vi "iHR550 Convert Axis.vi"(1 "iHR Current Values":T2={"iHR 550 Front Entrance"=0.0, "iHR550 Side Exit"=0.0, "iHR550 Wavelength"=897.9988, "iHR550 Exit Mirror"=2, "iHR550 Grating"="1", "Grating Index"=1} {"iHR550 Exit Mirror" items=["EntranceMirror", "ExitMirror", "Front", "Side"]}) -> (0 "Wavelengths (nm)":dbl[](array[numeric]))   [LabVIEW 2010]
uses:
  TypeDefs/iHR Current Values.ctl
  TypeDefs/iHR Instrument Parameters.ctl
panel:
  out "Tabellen-String":string
  out "l_p (nm)":dbl
  out "beta_lp (rad)":dbl
  out "H_Blp (mm)":dbl
  out "P_c":dbl
  out "beta_H (rad)":dbl
  out "beta_lc (rad)":dbl
  in  "Diffraction Order":i8=1
  in  "Grooves (1/mm)":i16[](array[numeric])=[1800, 600, 150]
  out "alpha_lc (rad)":dbl
  out "H_Blc (mm)":dbl
  out "L_H (mm)":dbl
  out "Inclination Angle (rad)":dbl
  out "Ebert Angle (rad)":dbl
  out "Pixel Width (mm)":dbl
  in  "iHR Instrument Parameters":T1={"Focal In (mm)"=546.0, "Focal Out (mm)"=568.72, "Pixel Width (µm)"=13.5, "Pixel Count"=2048, "Ebert Angle (°)"=6.498, "Inclination Angle (°)"=-2.35}
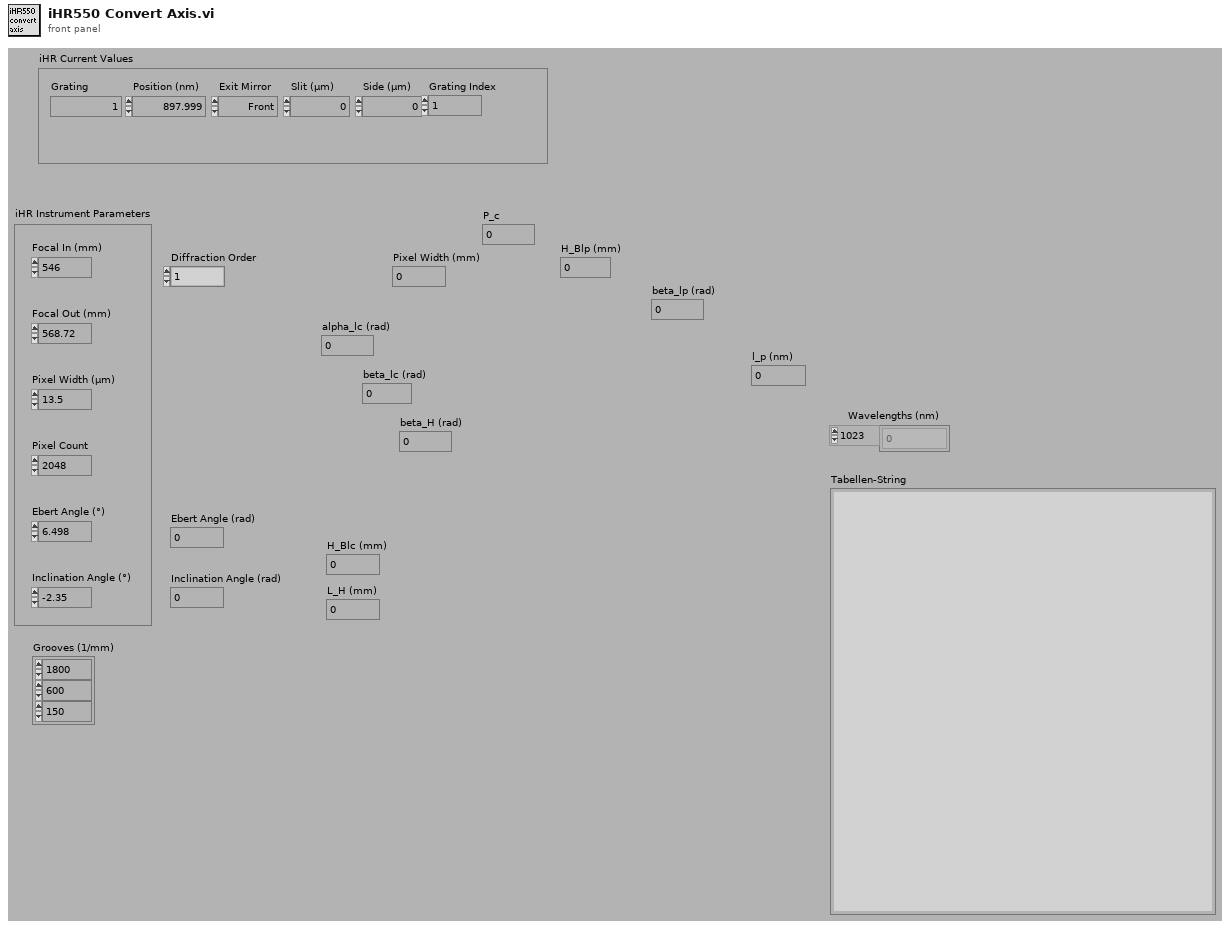
[diagram p1: front panel]
types:
  T1 = typedef "iHR Instrument Parameters.ctl" = cluster{"Focal In (mm)":dbl, "Focal Out (mm)":dbl, "Pixel Width (µm)":dbl, "Pixel Count":i16, "Ebert Angle (°)":dbl, "Inclination Angle (°)":dbl}
  T2 = typedef "iHR Current Values.ctl" = cluster{"iHR 550 Front Entrance":dbl, "iHR550 Side Exit":dbl, "iHR550 Wavelength":dbl, "iHR550 Exit Mirror":i32, "iHR550 Grating":string, "Grating Index":i32}
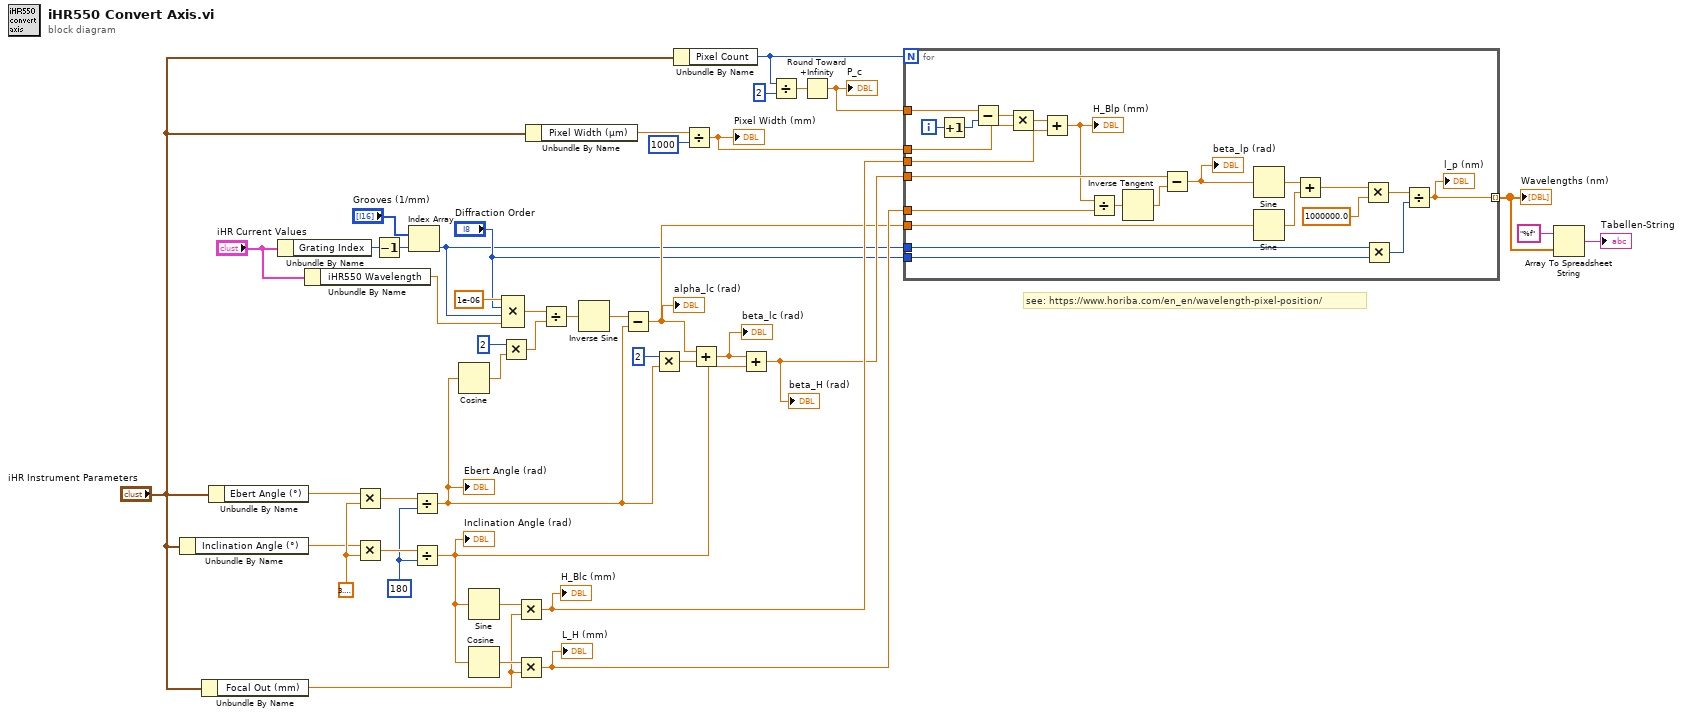
[diagram p0: block diagram]
diagram:
  w40 = i16 180 ("y")
  w42 = 3.141592653589793
  # "see: https://www.horiba.com/en_en/wavelength-pixel-position/"
  n1 = Unbundle By Name("iHR Instrument Parameters") -> ("Inclination Angle (°)"=w36:dbl)
  n2 = Unbundle By Name("iHR Instrument Parameters") -> ("Focal Out (mm)"=w32:dbl)
  n3 = Unbundle By Name("iHR Instrument Parameters") -> ("Ebert Angle (°)"=w37:dbl)
  n4 = Unbundle By Name("iHR Current Values") -> ("Grating Index"=w25:i32)
  n5 = Unbundle By Name("iHR Current Values") -> ("iHR550 Wavelength"=w20:dbl)
  n6 = Multiply(x=w37, y=w42) -> (x*y=w43:dbl)
  n7 = Multiply(x=w36, y=w42) -> (x*y=w41:dbl)
  n8 = Decrement(x=w25) -> (x-1=w24:i32)
  n9 = Index Array(array="Grooves (1/mm)", index=w24) -> (element=w4:i16)
  n10 = Divide(x=w43, y=w40) -> (x/y=w17:dbl)
  "Ebert Angle (rad)" <- w17
  n11 = Divide(x=w41, y=w40) -> (x/y=w15:dbl)
  "Inclination Angle (rad)" <- w15
  n12 = Cosine(x=w17) -> (cos(x)=w27:dbl)
  n13 = Sine(x=w15) -> (sin(x)=w33:dbl)
  n14 = Cosine(x=w15) -> (cos(x)=w34:dbl)
  n15 = Multiply(x=i8 2, y=w27) -> (x*y=w29:dbl)
  n16 = Compound Arithmetic op=MULTIPLY(1e-06 ("value"), "Diffraction Order", w4, w20) -> (w22:dbl)
  n17 = Multiply(x=w33, y=w32) -> (x*y=w14:dbl)
  "H_Blc (mm)" <- w14
  n18 = Multiply(x=w34, y=w32) -> (x*y=w7:dbl)
  "L_H (mm)" <- w7
  n19 = Unbundle By Name("iHR Instrument Parameters") -> ("Pixel Width (µm)"=w38:dbl)
  n20 = Divide(x=w22, y=w29) -> (x/y=w30:dbl)
  n21 = Inverse Sine(1:w30) -> (0:w31:dbl)
  n22 = Subtract(x=w31, y=w17) -> (x-y=w6:dbl)
  "alpha_lc (rad)" <- w6
  n23 = Multiply(x=i8 2, y=w17) -> (x*y=w18:dbl)
  n24 = Unbundle By Name("iHR Instrument Parameters") -> ("Pixel Count"=w13:i16)
  n25 = Divide(x=w38, y=i16 1000) -> (x/y=w9:dbl)
  "Pixel Width (mm)" <- w9
  n26 = Add(x=w6, y=w18) -> (x+y=w16:dbl)
  "beta_lc (rad)" <- w16
  n27 = Add(x=w16, y=w15) -> (x+y=w8:dbl)
  "beta_H (rad)" <- w8
  n28 = Divide(x=w13, y=i16 2) -> (x/y=w11:dbl)
  n29 = Round Toward +Infinity(x=w11) -> (ceil(x): smallest int >= x=w10:dbl)
  "P_c" <- w10
  n30 = for {
    N: w13 -> [_]
    tunnel: w14 -> [w65]
    tunnel: w10 -> [w62]
    tunnel: w9 -> [w60]
    tunnel: w8 -> [w58]
    tunnel: w7 -> [w55]
    tunnel: [w50] -> w1 mode=indexing
    tunnel: w6 -> [w48]
    tunnel: "Diffraction Order" -> [w45]
    tunnel: w4 -> [w44]
    i -> [w64]
    n31 = Increment(x=w64) -> (x+1=w63:i32)
    n32 = Subtract(x=w62, y=w63) -> (x-y=w61:dbl)
    n33 = Multiply(x=w61, y=w60) -> (x*y=w66:dbl)
    n34 = Add(x=w66, y=w65) -> (x+y=w56:dbl)
    "H_Blp (mm)" <- w56
    n35 = Divide(x=w56, y=w55) -> (x/y=w57:dbl)
    n36 = Inverse Tangent(1:w57) -> (0:w59:dbl)
    n37 = Subtract(x=w58, y=w59) -> (x-y=w49:dbl)
    "beta_lp (rad)" <- w49
    n38 = Sine(x=w49) -> (sin(x)=w47:dbl)
    n39 = Sine(x=w48) -> (sin(x)=w46:dbl)
    n40 = Add(x=w47, y=w46) -> (x+y=w53:dbl)
    n41 = Multiply(x=w53, y=1000000.0) -> (x*y=w51:dbl)
    n42 = Multiply(x=w44, y=w45) -> (x*y=w54:i16)
    n43 = Divide(x=w51, y=w54) -> (x/y=w50:dbl)
    "l_p (nm)" <- w50
  }
  "Wavelengths (nm)" <- w1
  n44 = Array To Spreadsheet String(array=w1, 3:"%f" ("Format-String")) -> (spreadsheet string=→"Tabellen-String":string)  [unwired: 1 in]
